vi "CreateTodayFolder.vi"(1 "data location":path=path "G:/Data") -> (0 "appended path":path)   [LabVIEW 2011]
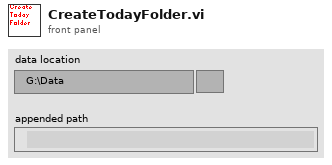
[diagram p1: front panel]
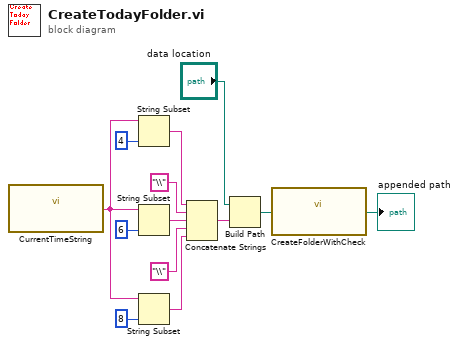
[diagram p0: block diagram]
diagram:
  n1 = call "CurrentTimeString.vi"() -> ("date/time string"=w10:string)
  n2 = String Subset(string=w10, length (rest)=4 ("length (rest)")) -> (substring=w9:string)  [unwired: 1 in]
  n3 = String Subset(string=w10, length (rest)=6 ("length (rest)")) -> (substring=w7:string)  [unwired: 1 in]
  n4 = String Subset(string=w10, length (rest)=8 ("length (rest)")) -> (substring=w5:string)  [unwired: 1 in]
  n5 = Concatenate Strings(w9, "\\" ("string"), w7, "\\" ("string"), w5) -> (w4:string)
  n6 = Build Path(base path="data location", name or relative path=w4) -> (appended path=w2:path)
  n7 = call "CreateFolderWithCheck.vi"("path"=w2) -> ("created path"=→"appended path":path)
